vi "main.vi"() -> ()   [LabVIEW 2013]
panel:
  in  "VI Ref":refnum<vi>
  in  "Tab Control":enum32{"Page 1", "Page 2"}(tab)
  out "String":string
  in  "Proximo":bool
  in  "Voltar":bool
  # "II Semana de Física Experimental"
  # "Criptografia Quântica"
  # "Laboratório de Óptica Quântica"
  # "UFRJ"
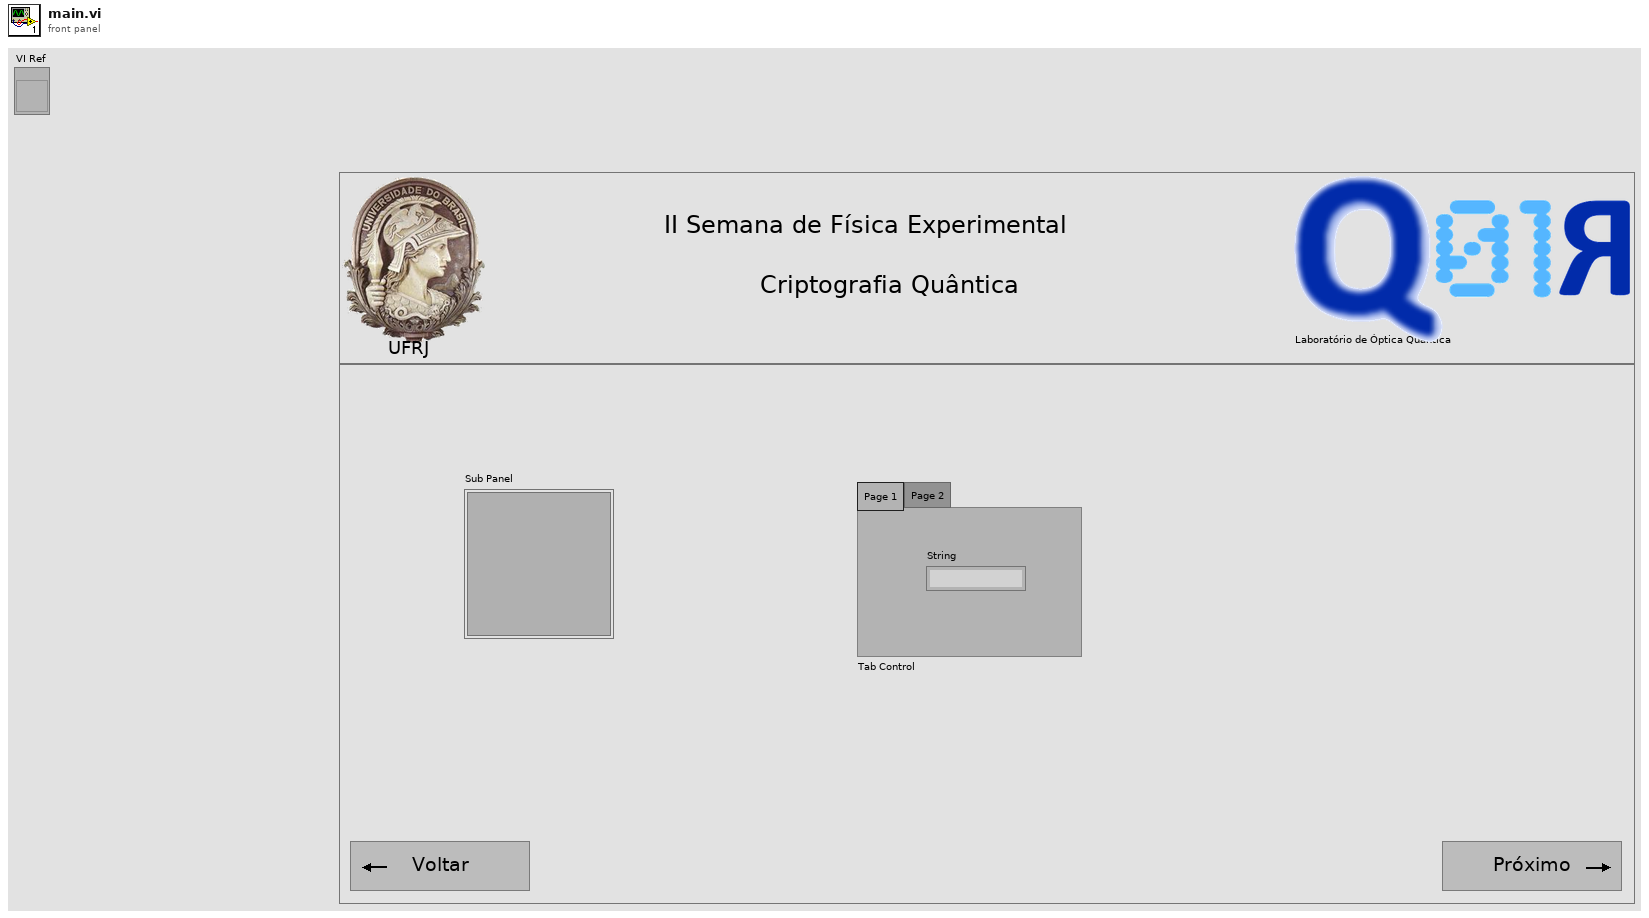
[diagram p1: front panel]
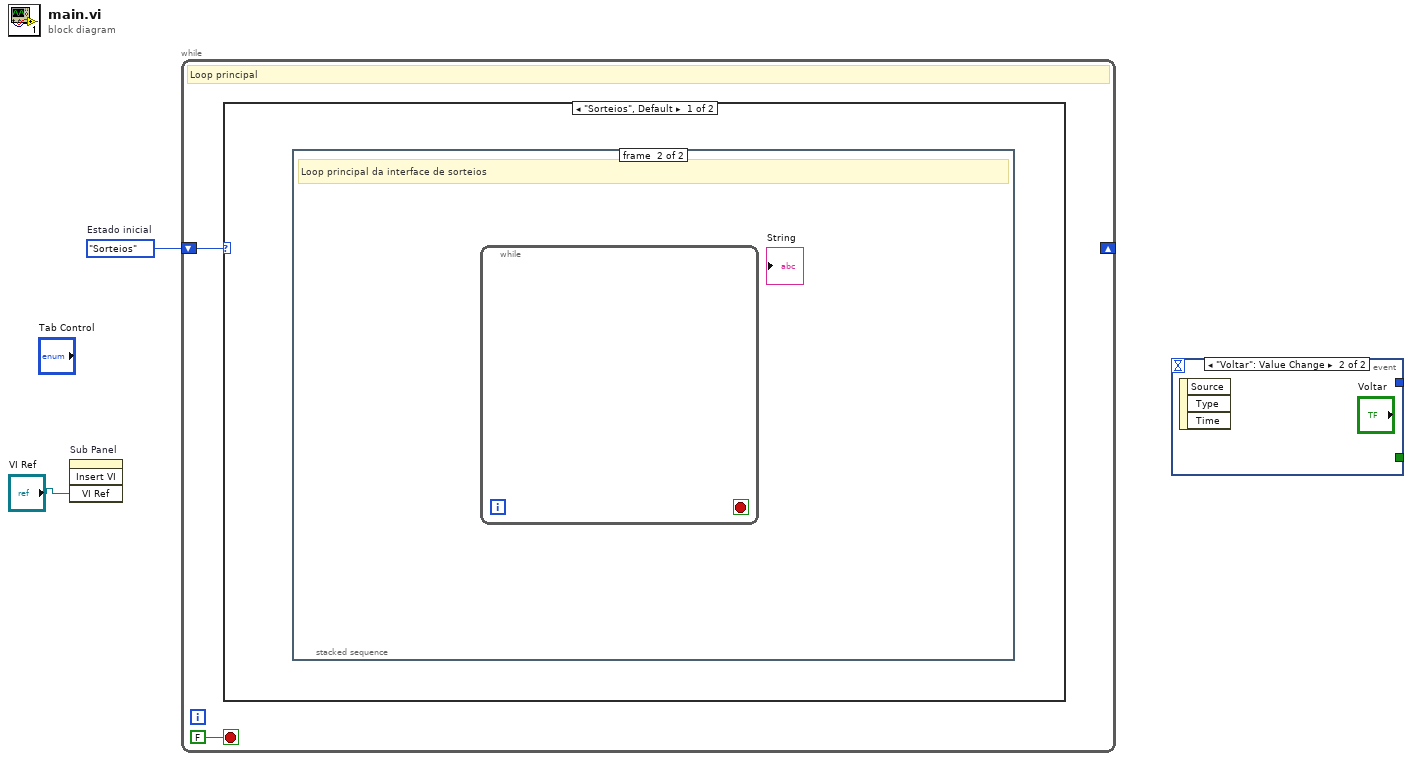
[diagram p0: block diagram]
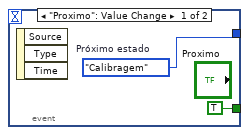
[diagram p2: hidden frame]
diagram:
  w2 = enum8{"Sorteios", "Calibragem"}."Sorteios"  # Estado inicial
  n1 = invoke on="Sub Panel" class="SubPanel" method="Insert VI"("VI Ref"="VI Ref") -> ()  [unwired: 3 in, 4 out]
  n2 = while {
    shift-right: _ -> [_]
    shift-left: w2 -> [w3]
    stop <- FALSE stop-if-true
    # "Loop principal"
    n3 = case shown="\"Sorteios\", Default" w3 {
      frame "Sorteios", Default {
        n4 = stacked-sequence {
          frame #0 {
            # "Inicializar interface de sorteios"
          }
          frame #1 {
            # "Loop principal da interface de sorteios"
            n5 = while {
              stop <- _ stop-if-true
            }
          }
        }
      }
      frame "Calibragem" {
      }
    }
  }
  n6 = event shown="[1] \"Voltar\": Value Change" {
    selector: _ -> [_ _]
    dyn-events: _ -> [_ _]
    timeout: _ -> [_ _]
    tunnel: [TRUE _] -> _
    tunnel: [w5 _] -> _
    event "Proximo": Value Change {
      w5 = enum8{"Sorteios", "Calibragem"}."Calibragem"  # Próximo estado
      n7 = event-data() -> ()  [unwired: 1 in, 3 out]
    }
    event "Voltar": Value Change {
      n8 = event-data() -> ()  [unwired: 1 in, 3 out]
    }
  }
